vi "(20) part 2 que.vi"() -> ()   [LabVIEW 2025]
uses:
  <vilib>/measure/NI_MABase.lvlib
panel:
  in  "Plot.Plot Color 2":u32(colorbox)
  in  "Plot.Plot Color":u32(colorbox)
  in  "Numeric":i32
  out "Waveform Graph":waveform(dbl)[](graph)
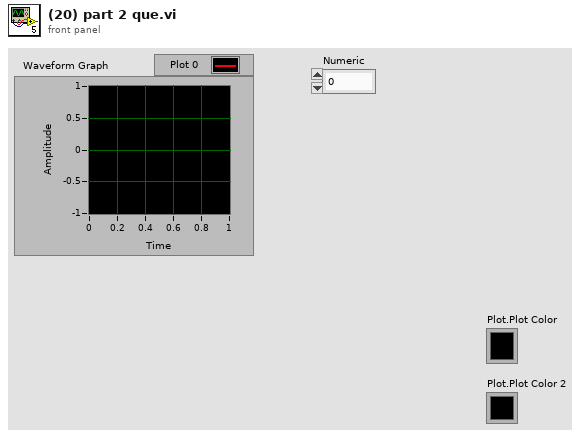
[diagram p1: front panel]
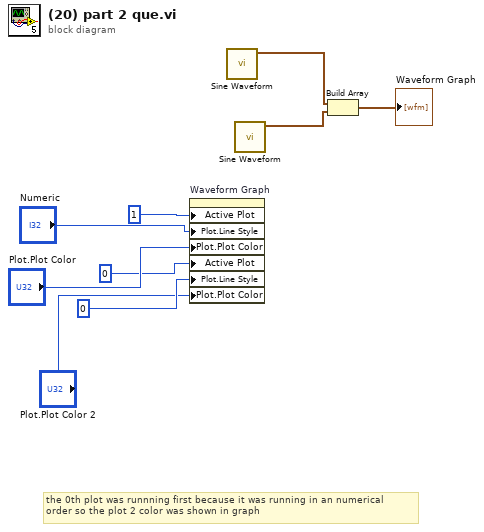
[diagram p0: block diagram]
diagram:
  # "the 0th plot was runnning first because it was running in an numerical \norder so the plot 2 color was shown in graph"
  n1 = property on="Waveform Graph" class="WFGraph (strict)"("Active Plot"=1, "Plot.Line Style"="Numeric", "Plot.Plot Color"="Plot.Plot Color", "Active Plot"=0, "Plot.Line Style"=0, "Plot.Plot Color"="Plot.Plot Color 2") -> ()  [unwired: 2 in, 2 out]
  n2 = call <vilib>:"Sine Waveform.vi"() -> ("signal out"=w3:waveform(dbl))  [unwired: 10 in, 1 out]
  n3 = call <vilib>:"Sine Waveform.vi"() -> ("signal out"=w4:waveform(dbl))  [unwired: 10 in, 1 out]
  n4 = Build Array(w3, w4) -> (→"Waveform Graph":waveform(dbl)[])
